vi "Get DDS Burst Period Ns.vi"(11 "channel_index":u8) -> (3 "function return":u64)   [LabVIEW 2021, in "vmmso.lvlib"]
doc: "DLL_API unsigned long long int WINAPI GetDDSBurstPeriodNs(unsigned char channel_index);"
uses:
  vmmso.lvlib
  vmmso.dll
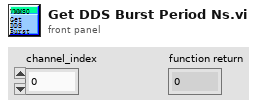
[diagram p1: front panel]
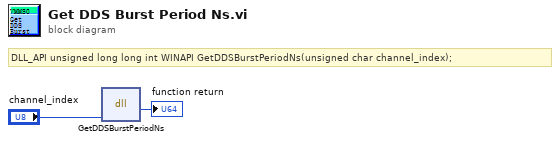
[diagram p0: block diagram]
diagram:
  # "DLL_API unsigned long long int WINAPI GetDDSBurstPeriodNs(unsigned char channel_index);"
  n1 = dll-call lib="D:/labviewdemo/LabviewDemo 21/vmmso/vmmso.*" fn="GetDDSBurstPeriodNs"("channel_index"="channel_index") -> (→"function return":u64)  [unwired: 4 in, 2 out]
